vi "Read code1.vi"(8 "error in (no error)":errorcluster, 11 "Child in":refnum<class "Child.lvclass">) -> (0 "error out":errorcluster, 2 "code1":dbl, 3 "Child out":refnum<class "Child.lvclass">)   [LabVIEW 2021, in "Child.lvclass"]
uses:
  Child.lvclass
  Child.lvclass/Child.ctl
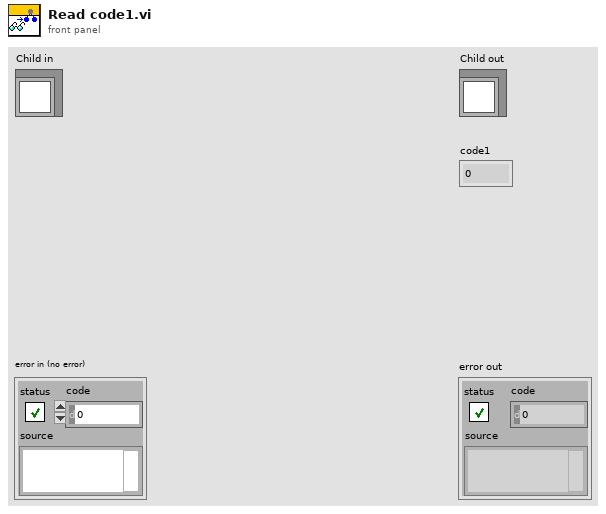
[diagram p1: front panel]
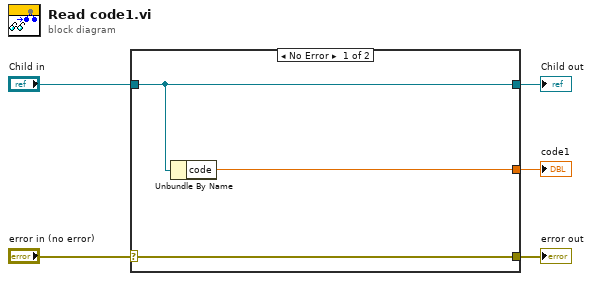
[diagram p0: block diagram]
diagram:
  n1 = case shown="No Error" "error in (no error)" {
    selector: "error in (no error)" -> [w8 w9]
    tunnel: [w8 w9] -> w4
    tunnel: [w7 w10] -> w2
    tunnel: "Child in" -> [w7 w10]
    tunnel: [w6 _] -> w1
    frame No Error {
      n2 = Unbundle By Name(w7) -> ("code"=w6:dbl)
    }
    frame Error {
    }
  }
  "error out" <- w4
  "Child out" <- w2
  "code1" <- w1
